vi "Read Results from processing.vi"(8 "error in":errorcluster, 11 "ScaleAndLimitModule runtime in":refnum<class "ScaleAndLimitModule runtime.lvclass">) -> (0 "error out":errorcluster, 2 "Results from processing":T1, 3 "ScaleAndLimitModule runtime out":refnum<class "ScaleAndLimitModule runtime.lvclass">)   [LabVIEW 2017, in "ScaleAndLimitModule runtime.lvclass"]
uses:
  ScaleAndLimitModule runtime.lvclass
  configuration/result data indices.ctl
  ScaleAndLimitModule runtime.lvclass/ScaleAndLimitModule runtime.ctl
  configuration/ScaleAndLimitModule configuration.lvclass
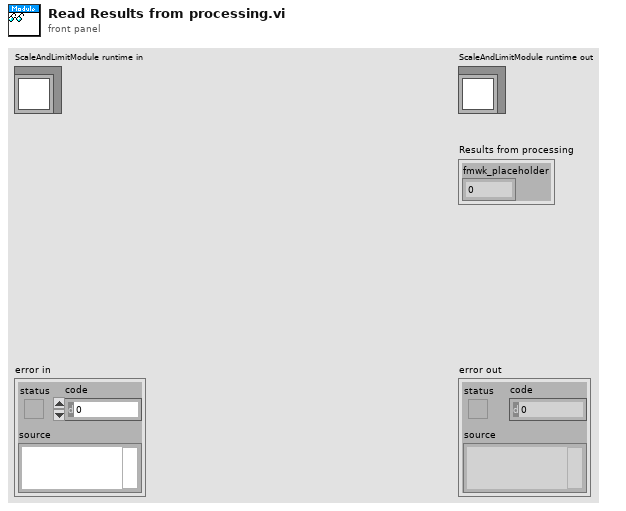
[diagram p1: front panel]
types:
  T1 = typedef "ScaleAndLimitModule configuration.lvclass/result data indices.ctl" = cluster{"fmwk_placeholder":i32}
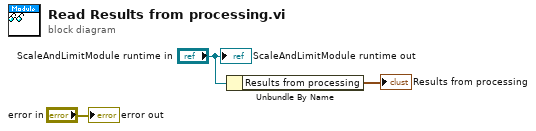
[diagram p0: block diagram]
diagram:
  n1 = Unbundle By Name("ScaleAndLimitModule runtime in") -> ("Results from processing"=→"Results from processing":T1)
  "error out" <- "error in"
  "ScaleAndLimitModule runtime out" <- "ScaleAndLimitModule runtime in"
